vi "S19 Convert File to Cluster Array.vi"(8 "error in":errorcluster, 11 "base path":path) -> (0 "Error Out":errorcluster, 1 "Address Min":u32 format="%.0x", 2 "Address Max":u32 format="%.0x", 3 "数组":T1(array[cluster]) {"Address" format="%x"; "Data" format="%x"; "CheckSUM" format="%x"})   [LabVIEW 2018]
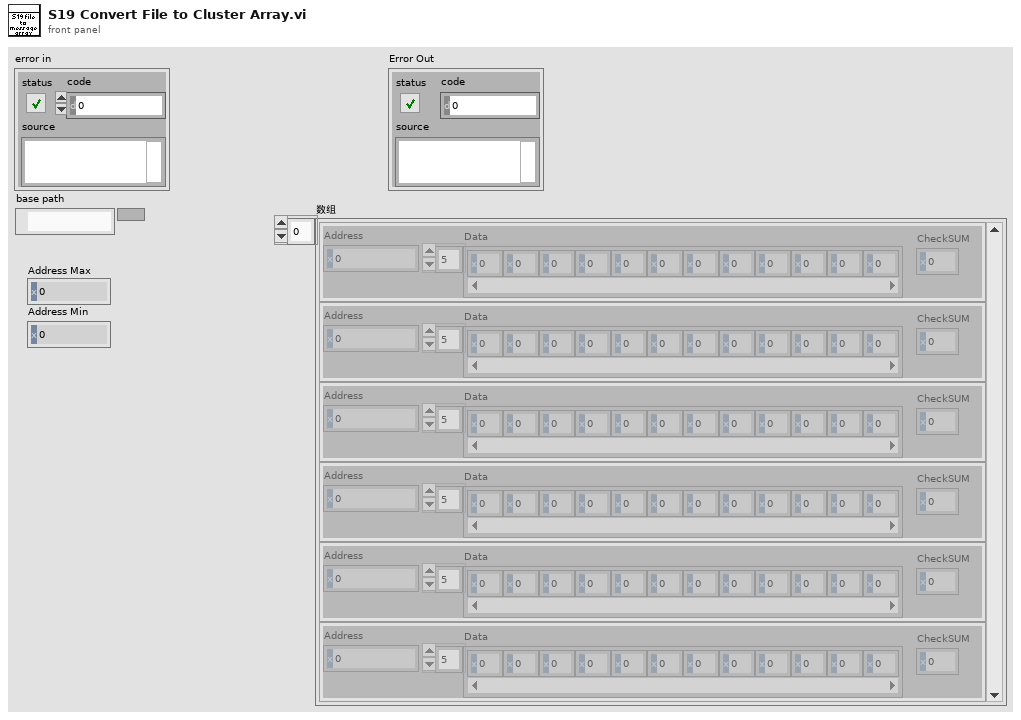
[diagram p1: front panel]
types:
  T1 = cluster{"Address":u32, "Data":u8[], "CheckSUM":u32}[]
  T2 = cluster{"Address":u32, "Data":u8[], "CheckSUM":u32}
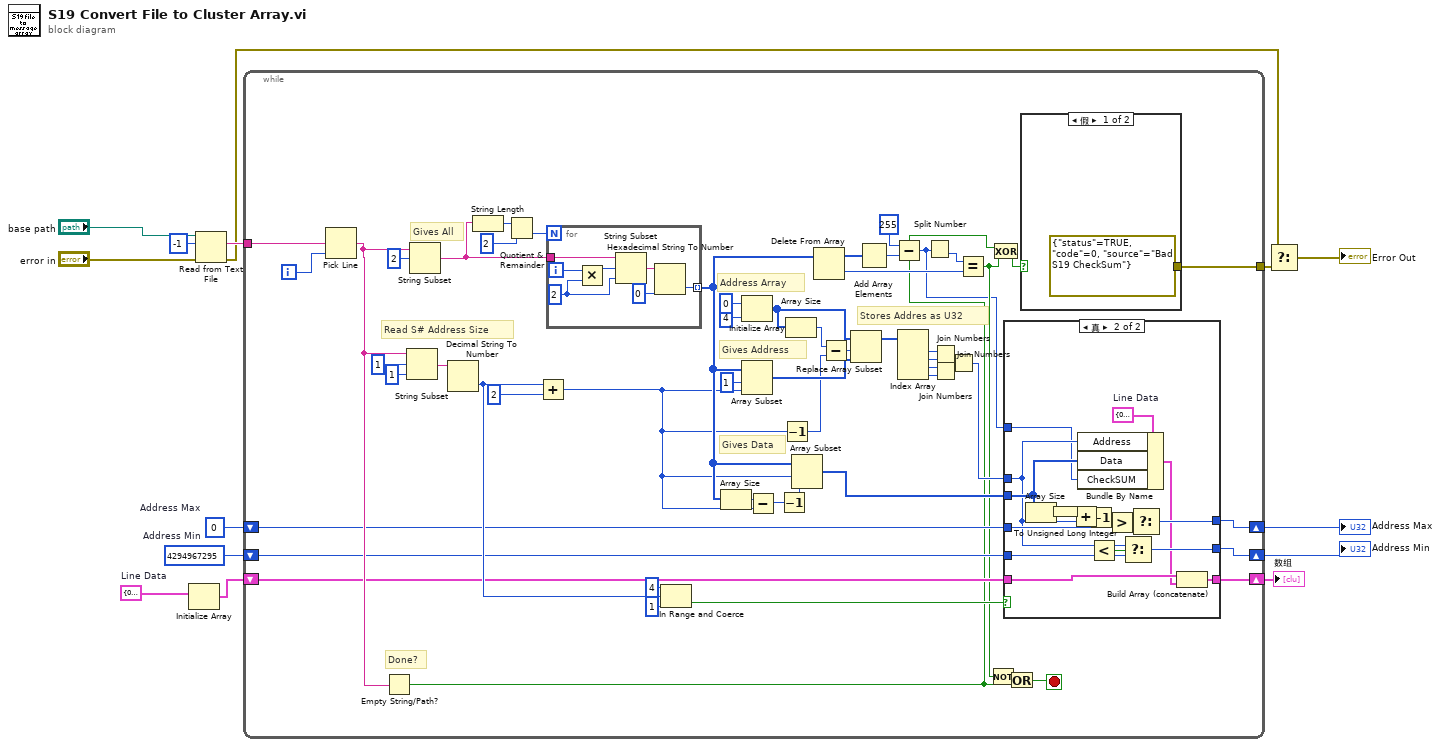
[diagram p0: block diagram]
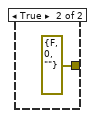
[diagram p3: hidden frame]
diagram:
  w2 = T2 {"Address"=0, "Data"=[], "CheckSUM"=0}  # Line Data
  w9 = u32 4294967295  # Address Min
  w10 = u32 0  # Address Max
  n1 = Initialize Array(w2) -> (w11:T1)  [unwired: 1 in]
  n2 = Read from Text File(file (use dialog)="base path", count=-1, error in="error in") -> (text=w12:string, error out=w7:errorcluster)  [unwired: 1 in, 2 out]
  n3 = while {
    tunnel: w12 -> [w70]
    shift-right: [w27] -> w1
    shift-left: w11 -> [w32]
    shift-right: [w29] -> w4
    shift-left: w10 -> [w31]
    shift-right: [w28] -> w3
    shift-left: w9 -> [w30]
    tunnel: [w26] -> w6
    i -> [w69]
    stop <- w58 stop-if-true
    # "Gives Data"
    # "Stores Addres as U32"
    # "Address Array"
    # "Gives Address"
    # "Done?"
    # "Gives All"
    # "Read S# Address Size"
    n4 = Pick Line(multi-line string=w70, line index=w69) -> (output string=w62:string)  [unwired: 1 in]
    n5 = Empty String/Path?(string/path=w62) -> (empty?=w20:bool)
    n6 = String Subset(string=w62, offset (0)=1, length (rest)=1 ("length (rest)")) -> (substring=w66:string)
    n7 = String Subset(string=w62, offset (0)=2) -> (substring=w23:string)  [unwired: 1 in]
    n8 = Decimal String To Number(string=w66) -> (number=w50:i32)  [unwired: 2 in, 1 out]
    n9 = String Length(string=w23) -> (length=w61:i32)
    n10 = Quotient & Remainder(x=w61, y=2) -> (floor(x/y)=w59:i32)  [unwired: 1 out]
    n11 = Add(x=w50, y=2) -> (x+y=w18:i32)
    n12 = for {
      N: w59 -> [_]
      tunnel: w23 -> [w99]
      tunnel: [w94] -> w36 mode=indexing
      i -> [w98]
      w96 = 2 ("x")
      n13 = Multiply(x=w98, y=w96) -> (x*y=w97:i32)
      n14 = String Subset(string=w99, offset (0)=w97, length (rest)=w96) -> (substring=w95:string)
      n15 = Hexadecimal String To Number(string=w95, default (0uL)=u8 0 ("default (0 U32)")) -> (number=w94:u8)  [unwired: 1 in, 1 out]
    }
    n16 = In Range and Coerce(upper limit=4, x=w50, lower limit=1) -> (In Range?=w35:bool)  [unwired: 1 out]
    n17 = Array Size(array=w36) -> (size(s)=w19:i32)
    n18 = Initialize Array(u8 0 ("index"), 4 ("dimension size")) -> (w47:u8[])
    n19 = Array Subset(array=w36, index=1, length=w18) -> (w37:u8[])
    n20 = Subtract(x=w19, y=w18) -> (x-y=w17:i32)
    n21 = Decrement(x=w17) -> (x-1=w16:i32)
    n22 = Decrement(x=w18) -> (x-1=w24:i32)
    n23 = Array Size(array=w47) -> (size(s)=w45:i32)
    n24 = Array Subset(array=w36, index=w18, length=w16) -> (w33:u8[])
    n25 = Delete From Array(array=w36) -> (deleted portion=w53:u8, array with subset deleted=w57:u8[])  [unwired: 2 in]
    n26 = Subtract(x=w45, y=w24) -> (x-y=w46:i32)
    n27 = Replace Array Subset(array=w47, new element=w37, index=w46) -> (w44:u8[])
    n28 = Add Array Elements(numeric array=w57) -> (sum=w54:u8)
    n29 = Subtract(x=u8 255, y=w54) -> (x-y=w15:u8)
    n30 = Index Array(array=w44) -> (element #1=w41:u8, element #2=w40:u8, element #3=w39:u8, element #4=w38:u8)  [unwired: 4 in]
    n31 = Split Number(x=w15) -> (lo(x)=w56:u8)  [unwired: 1 out]
    n32 = Join Numbers(hi=w41, lo=w40) -> ((hi.lo)=w43:u16)
    n33 = Join Numbers(hi=w39, lo=w38) -> ((hi.lo)=w42:u16)
    n34 = Join Numbers(hi=w43, lo=w42) -> ((hi.lo)=w34:u32)
    n35 = Equal?(x=w56, y=w53) -> (x = y?=w22:bool)
    n36 = Not(x=w22) -> (.not. x?=w25:bool)
    n37 = Exclusive Or(1:w22, 2:w20) -> (0:w21:bool)
    n38 = case shown="真" w35 {
      tunnel: w34 -> [_ w78]
      tunnel: w33 -> [_ w80]
      tunnel: w32 -> [w71 w83]
      tunnel: w31 -> [w73 w88]
      tunnel: w30 -> [w72 w86]
      tunnel: [w73 w85] -> w29
      tunnel: [w72 w84] -> w28
      tunnel: [w71 w81] -> w27
      tunnel: w15 -> [_ w74]
      frame False {
      }
      frame True {
        w89 = T2 {"Address"=0, "Data"=[], "CheckSUM"=0}  # Line Data
        n39 = Array Size(array=w80) -> (size(s)=w79:i32)
        n40 = To Unsigned Long Integer(number=w79) -> (unsigned 32bit integer=w76:u32)
        n41 = Add(x=w76, y=w78) -> (x+y=w77:u32)
        n42 = Bundle By Name(cluster=w89, "Address"=w78, "Data"=w80, "CheckSUM"=w74) -> (w82:T2)
        n43 = Decrement(x=w77) -> (x-1=w75:u32)
        n44 = Less?(x=w78, y=w86) -> (x < y?=w87:bool)
        n45 = Greater?(x=w75, y=w88) -> (0:w90:bool)
        n46 = Select(t=w78, s=w87, f=w86) -> (s? t:f=w84:u32)
        n47 = Select(t=w75, s=w90, f=w88) -> (s? t:f=w85:u32)
        n48 = Build Array (concatenate)(w83, w82) -> (w81:T1)
      }
    }
    n49 = Or(x=w25, y=w20) -> (x .or. y?=w58:bool)
    n50 = case shown="假" w21 {
      tunnel: [errorcluster {"status"=TRUE, "code"=0, "source"="Bad S19 CheckSum"} ("error constant") errorcluster {"status"=FALSE, "code"=0, "source"=""} ("error constant")] -> w26
      frame False {
      }
      frame True {
      }
    }
  }
  "Address Max" <- w4
  "Address Min" <- w3
  "数组" <- w1
  n51 = Select(t=w7, s=w7, f=w6) -> (s? t:f=→"Error Out":errorcluster)
